vi "pmu_Buffer Reporting Data.vi"(7 "reset? (F)":bool, 8 "buffer length":i32, 10 "GPS information":T3[](array[typedef]), 11 "raw data":T2(array[cluster])) -> (0 "empty?":bool, 2 "reporting GPS information":T3, 3 "reporting raw data":T1)   [LabVIEW 2013, in "NI_EP_PMU.lvlib"]
uses:
  <vilib>/addons/Electrical Power/PMU/NI_EP_PMU.lvlib
  <vilib>/addons/Electrical Power/PMU/Common/Controls/pmu_GPS Info.ctl
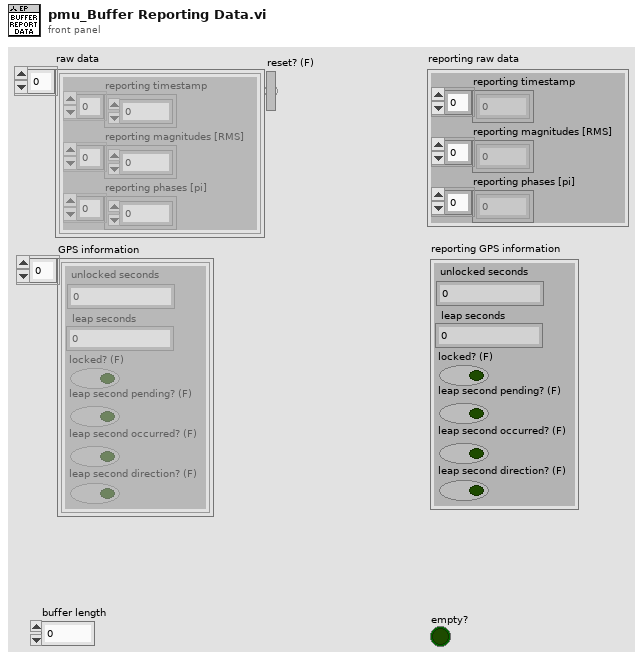
[diagram p1: front panel]
types:
  T1 = cluster{"reporting timestamp":dbl[], "reporting magnitudes [RMS]":dbl[], "reporting phases [pi]":dbl[]}
  T2 = cluster{"reporting timestamp":dbl[], "reporting magnitudes [RMS]":dbl[], "reporting phases [pi]":dbl[]}[]
  T3 = typedef "NI_EP_PMU.lvlib/pmu_GPS Info.ctl" = cluster{"unlocked seconds":u32, "leap seconds":i8, "locked? (F)":bool, "leap second pending? (F)":bool, "leap second occurred? (F)":bool, "leap second direction? (F)":bool}
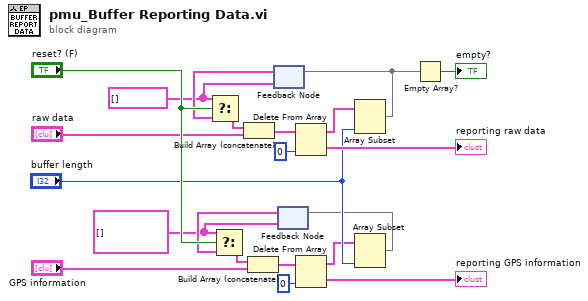
[diagram p0: block diagram]
diagram:
  w8 = T2 [] ("raw data")
  w7 = T3[] [] ("t")
  n1 = feedback #1(w8) -> (w16:T2)
  n2 = Select(t=w8, s="reset? (F)", f=w16) -> (s? t:f=w19:T2)
  n3 = Build Array (concatenate)(w19, "raw data") -> (w13:T2)
  n4 = feedback #2(w7) -> (w15:T3[])
  n5 = Select(t=w7, s="reset? (F)", f=w15) -> (s? t:f=w21:T3[])
  n6 = Build Array (concatenate)(w21, "GPS information") -> (w10:T3[])
  n7 = Delete From Array(array=w13, index=0) -> (deleted portion=→"reporting raw data":T1, array with subset deleted=w4:T2)  [unwired: 1 in]
  n8 = Delete From Array(array=w10, index=0) -> (deleted portion=→"reporting GPS information":T3, array with subset deleted=w5:T3[])  [unwired: 1 in]
  n9 = Array Subset(array=w4, length="buffer length") -> (w2:T2)  [unwired: 1 in]
  n10 = feedback-in #1(w2) -> ()
  n11 = Array Subset(array=w5, length="buffer length") -> (w3:T3[])  [unwired: 1 in]
  n12 = feedback-in #2(w3) -> ()
  n13 = Empty Array?(array=w2) -> (empty?=→"empty?":bool)
